vi "TilePositionToIndex.vi"(11 "Position":T1) -> (3 "Numeric":u16)   [LabVIEW 2019, in "RT_Game.lvlib" / "Engine.lvclass"]
uses:
  Engine.lvclass
  Game/Coordinate.ctl
  Game/Game.lvclass
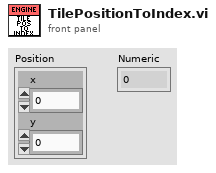
[diagram p1: front panel]
types:
  T1 = typedef "RT_Game.lvlib/Game.lvclass/Coordinate.ctl" = cluster{"x":dbl, "y":dbl}
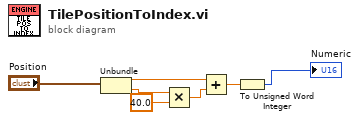
[diagram p0: block diagram]
diagram:
  n1 = Unbundle("Position") -> ("x"=w4:dbl, "y"=w2:dbl)
  n2 = Multiply(x=w2, y=40.0) -> (x*y=w5:dbl)
  n3 = Add(x=w4, y=w5) -> (x+y=w6:dbl)
  n4 = To Unsigned Word Integer(number=w6) -> (unsigned 16bit integer=→"Numeric":u16)
